vi "RUN ARM MACRO ARRAY.vi"(0 "LEFT or RIGHT":string, 1 "invert Climber sensor?":bool, 2 "invert ANGLE sensor?":bool, 5 "element of ARRAY ROW":T2 {"Angle"."speed" min=0.0 max=1.0 format="%_3g"; "Angle"."ARM ANGLE (deg)" format="%.3g"; "Climber"."CLIMBER STROKE (in)" format="%_5g"; "Climber"."speed" min=0.0 max=1.0 format="%_3g"}, 9 "Climber PID gains":T1={"proportional gain (Kc)"=0.05, "integral time (Ti, min)"=0.05, "derivative time (Td, min)"=0.006} {"derivative time (Td, min)" format="%.3f"; "integral time (Ti, min)" format="%.3f"; "proportional gain (Kc)" format="%.6f"}, 11 "Angle PID gains":T1={"proportional gain (Kc)"=1.0, "integral time (Ti, min)"=0.0, "derivative time (Td, min)"=0.0} {"derivative time (Td, min)" format="%.3f"; "integral time (Ti, min)" format="%.3f"; "proportional gain (Kc)" format="%.6f"}, 13 "convert inches travel to degrees from vertical":dbl=4.96493) -> ()   [LabVIEW 2020]
uses:
  ctrl ARM MACRO ENTRY.ctl
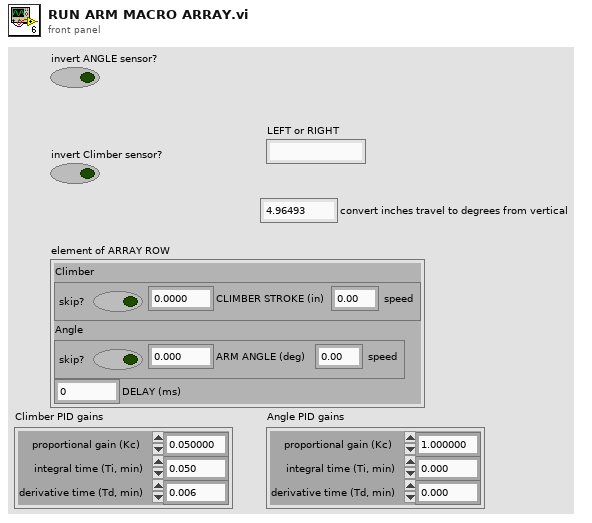
[diagram p1: front panel]
types:
  T1 = cluster{"proportional gain (Kc)":dbl, "integral time (Ti, min)":dbl, "derivative time (Td, min)":dbl}
  T2 = typedef "ctrl ARM MACRO ENTRY.ctl" = cluster{"Climber":cluster{"skip?":bool, "CLIMBER STROKE (in)":dbl, " speed":dbl}, "Angle":cluster{"skip?":bool, "ARM ANGLE (deg)":dbl, " speed":dbl}, "DELAY (ms)":u32}
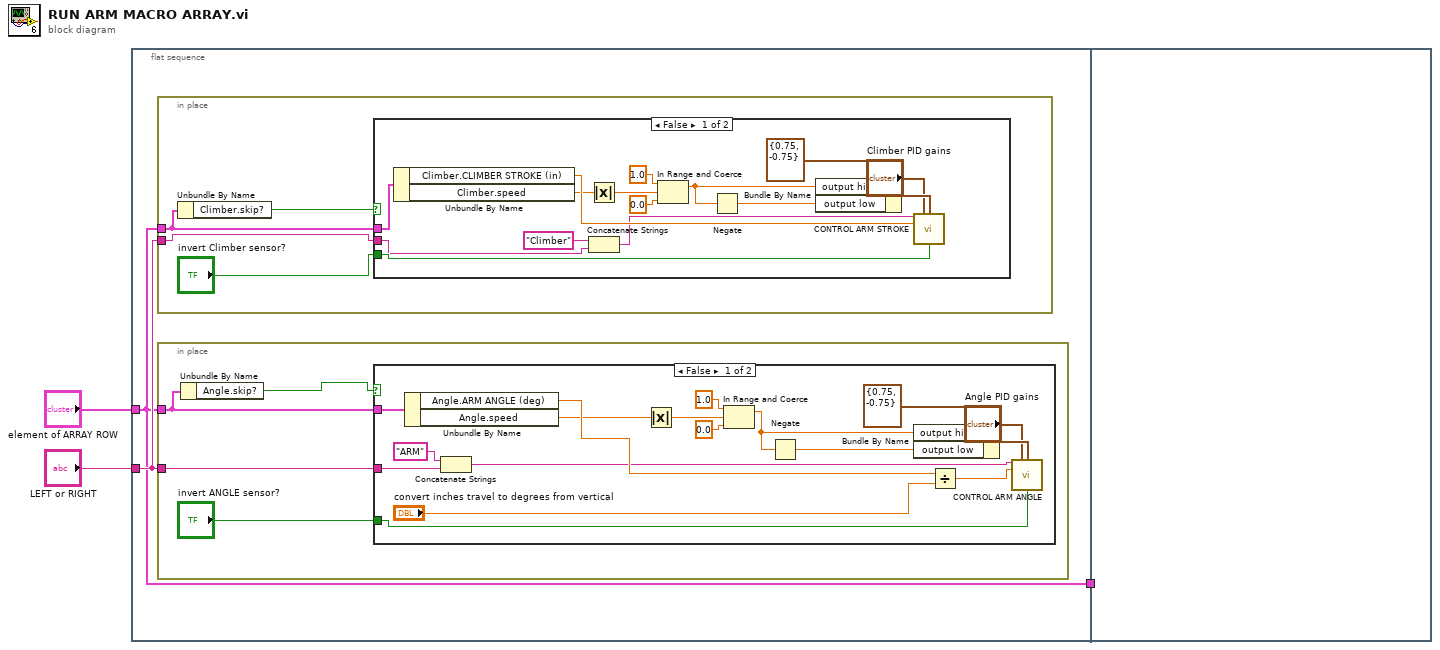
[diagram p0: block diagram]
diagram:
  n1 = flat-sequence {
    tunnel: "LEFT or RIGHT" -> [w5]
    tunnel: "element of ARRAY ROW" -> [w4]
    tunnel: [w4] -> w1
    tunnel: w1 -> [_]
    frame #0 {
      n2 = in-place {
        in-place-border: w5 -> [w9]
        in-place-border: w4 -> [w8]
        n3 = Unbundle By Name(w8) -> ("Climber.skip?"=w7:bool)
        n4 = case shown="False" w7 {
          tunnel: w8 -> [w23 _]
          tunnel: "invert Climber sensor?" -> [w17 _]
          tunnel: w9 -> [w15 _]
          frame False {
            n5 = Unbundle By Name(w23) -> ("Climber.CLIMBER STROKE (in)"=w22:dbl, "Climber.speed"=w20:dbl)
            n6 = Absolute Value(x=w20) -> (abs(x)=w14:dbl)
            n7 = Concatenate Strings("Climber", w15) -> (w16:string)
            n8 = In Range and Coerce(upper limit=1.0, x=w14, lower limit=0.0) -> (coerced(x)=w13:dbl)  [unwired: 1 out]
            n9 = Negate(x=w13) -> (-x=w19:dbl)
            n10 = Bundle By Name(cluster=cluster{"output high":dbl, "output low":dbl} {"output high"=0.75, "output low"=-0.75} ("output range"), "output high"=w13, "output low"=w19) -> (w18:cluster{"output high":dbl, "output low":dbl})
            n11 = call "CONTROL ARM STROKE.vi"("refnum name"=w16, "PID gains"="Climber PID gains", "output range"=w18, "setpoint (in)"=w22, "invert sensor?"=w17) -> ()  [unwired: 9 in, 2 out]
          }
          frame True {
          }
        }
      }
      n12 = in-place {
        in-place-border: w5 -> [w28]
        in-place-border: w4 -> [w27]
        n13 = Unbundle By Name(w27) -> ("Angle.skip?"=w25:bool)
        n14 = case shown="False" w25 {
          tunnel: w27 -> [w44 _]
          tunnel: "invert ANGLE sensor?" -> [w38 _]
          tunnel: w28 -> [w36 _]
          frame False {
            n15 = Unbundle By Name(w44) -> ("Angle.ARM ANGLE (deg)"=w43:dbl, "Angle.speed"=w41:dbl)
            n16 = Concatenate Strings("ARM", w36) -> (w37:string)
            n17 = Absolute Value(x=w41) -> (abs(x)=w35:dbl)
            n18 = In Range and Coerce(upper limit=1.0, x=w35, lower limit=0.0) -> (coerced(x)=w34:dbl)  [unwired: 1 out]
            n19 = Negate(x=w34) -> (-x=w40:dbl)
            n20 = Bundle By Name(cluster=cluster{"output high":dbl, "output low":dbl} {"output high"=0.75, "output low"=-0.75} ("output range"), "output high"=w34, "output low"=w40) -> (w39:cluster{"output high":dbl, "output low":dbl})
            n21 = Divide(x=w43, y="convert inches travel to degrees from vertical") -> (x/y=w31:dbl)
            n22 = call "CONTROL ARM ANGLE.vi"("refnum name"=w37, "PID gains"="Angle PID gains", "output range"=w39, "setpoint (in)"=w31, "invert sensor?"=w38) -> ()  [unwired: 9 in, 2 out]
          }
          frame True {
          }
        }
      }
    }
    frame #1 {
    }
  }
